vi "Test.vi"   [LabVIEW 2013]
doc: "This VI is called when test mode begins, and will automatically be terminated when it ends. You can add manual or automatic tests and invoke them from the dashboard."
uses:
  Robot Global Data.vi
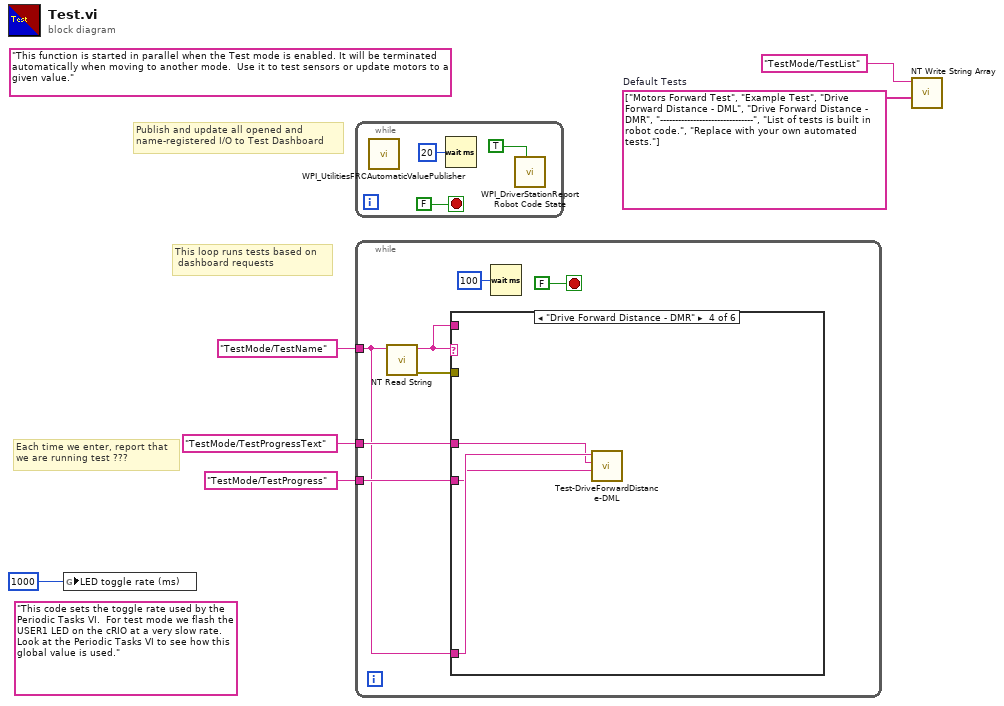
[diagram p0: block diagram]
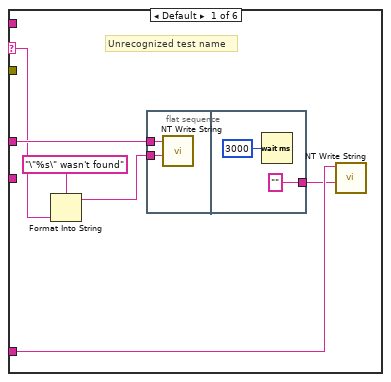
[diagram p2: hidden frame]
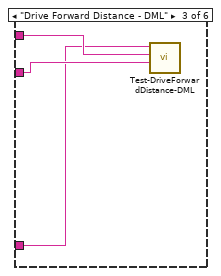
[diagram p4: hidden frame]
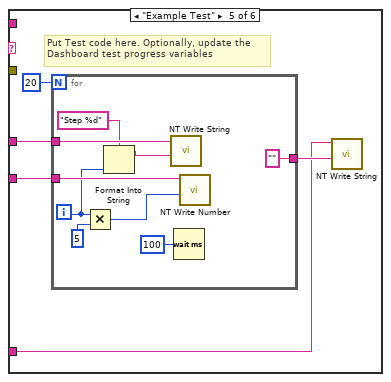
[diagram p5: hidden frame]
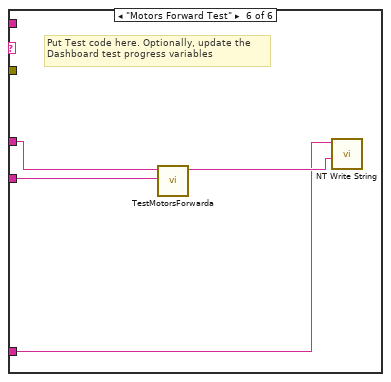
[diagram p6: hidden frame]
diagram:
  w2 = string[] ["Motors Forward Test", "Example Test", "Drive Forward Distance - DML", "Drive Forward Distance - DMR", "-------------------------------", "List of tests is built in robot code.", "Replace with your own automated tests."]  # Default Tests
  (unwired) "This code sets the toggle rate used by the Periodic Tasks VI.  For test mode we flash the USER1 LED on the cRIO at a very slow rate.  Look at the Periodic Tasks VI to see how this global value is used."
  (unwired) "This function is started in parallel when the Test mode is enabled. It will be terminated automatically when moving to another mode.  Use it to test sensors or update motors to a given value."
  # "This loop runs tests based on \n dashboard requests"
  # "Publish and update all opened and\nname-registered I/O to Test Dashboard"
  # "Each time we enter, report that\nwe are running test ???"
  n1 = global write "Robot Global Data.vi" "LED toggle rate (ms)"(u32 1000 ("LED ms toggle rate")) -> ()
  n2 = while {
    stop <- FALSE stop-if-true
    n3 = call <vilib>:"WPI_UtilitiesFRCAutomaticValuePublisher.vi"() -> ()  [unwired: 12 in]
    n4 = Wait (ms)(milliseconds to wait=u32 20) -> ()  [unwired: 1 out]
    n5 = call <vilib>:"WPI_DriverStationReport Robot Code State.vi"("Test"=TRUE ("Autonomous")) -> ()  [unwired: 10 in, 1 out]
  }
  n6 = while {
    tunnel: "TestMode/TestName" ("Name") -> [w11]
    tunnel: "TestMode/TestProgressText" ("Name") -> [w14]
    tunnel: "TestMode/TestProgress" ("Name") -> [w13]
    stop <- FALSE stop-if-true
    n7 = call <vilib>:"NT Read String.vi"("Name"=w11) -> ("error out"=w10:errorcluster, "String"=w12:string)  [unwired: 9 in]
    n8 = case shown="\"Drive Forward Distance - DMR\"" w12 {
      selector: w12 -> [w21 _ _ _ _ _]
      tunnel: w11 -> [w18 _ w27 w32 w33 w47]
      tunnel: w14 -> [w22 _ w29 w31 w36 w49]
      tunnel: w13 -> [_ _ w28 w30 w37 w50]
      tunnel: w12 -> [_ _ _ _ _ _]
      tunnel: w10 -> [_ _ _ _ _ _]
      frame Default {
        # "Unrecognized test name"
        n9 = Format Into String(format string="\"%s\" wasn't found" ("Name"), w21) -> (resulting string=w20:string)  [unwired: 2 in, 1 out]
        n10 = flat-sequence {
          tunnel: w22 -> [w23]
          tunnel: w20 -> [w24]
          tunnel: ["" ("Name")] -> w17
          frame #0 {
            n11 = call <vilib>:"NT Write String.vi"("String"=w24, "Name"=w23) -> ()  [unwired: 9 in, 1 out]
          }
          frame #1 {
            n12 = Wait (ms)(milliseconds to wait=u32 3000) -> ()  [unwired: 1 out]
          }
        }
        n13 = call <vilib>:"NT Write String.vi"("String"=w17, "Name"=w18) -> ()  [unwired: 9 in, 1 out]
      }
      frame "" {
        # "No test to run"
      }
      frame "Drive Forward Distance - DML" {
        n14 = call "Test-DriveForwardDistance-DML.vi"("TestProgress NT"=w28, "TestProgressText NT"=w29, "TestName NT"=w27) -> ()  [unwired: 9 in]
      }
      frame "Drive Forward Distance - DMR" {
        n15 = call "Test-DriveForwardDistance-DML.vi"("TestProgress NT"=w30, "TestProgressText NT"=w31, "TestName NT"=w32) -> ()  [unwired: 9 in]
      }
      frame "Example Test" {
        # "Put Test code here. Optionally, update the\nDashboard test progress variables"
        n16 = for {
          N: 20 -> [_]
          tunnel: w37 -> [w46]
          tunnel: w36 -> [w44]
          tunnel: ["" ("String")] -> w34
          i -> [w41]
          n17 = Multiply(x=w41, y=u32 5 ("milliseconds to wait")) -> (x*y=w42:u32)
          n18 = Format Into String(format string="Step %d", w41) -> (resulting string=w39:string)  [unwired: 2 in, 1 out]
          n19 = call <vilib>:"NT Write String.vi"("String"=w39, "Name"=w44) -> ()  [unwired: 9 in, 1 out]
          n20 = Wait (ms)(milliseconds to wait=u32 100) -> ()  [unwired: 1 out]
          n21 = call <vilib>:"NT Write Number.vi"("Numeric"=w42, "Name"=w46) -> ()  [unwired: 9 in, 1 out]
        }
        n22 = call <vilib>:"NT Write String.vi"("String"=w34, "Name"=w33) -> ()  [unwired: 9 in, 1 out]
      }
      frame "Motors Forward Test" {
        # "Put Test code here. Optionally, update the\nDashboard test progress variables"
        n23 = call "TestMotorsForwarda.vi"("Name 2"=w50, "Name"=w49) -> ("String"=w48:string)  [unwired: 9 in]
        n24 = call <vilib>:"NT Write String.vi"("String"=w48, "Name"=w47) -> ()  [unwired: 9 in, 1 out]
      }
    }
    n25 = Wait (ms)(milliseconds to wait=u32 100) -> ()  [unwired: 1 out]
  }
  n26 = call <vilib>:"NT Write String Array.vi"("String Array"=w2, "Name"="TestMode/TestList") -> ()  [unwired: 9 in, 1 out]
